vi "Cycle_History_Parse.vi"(10 "Data":string, 11 "Cycle diag in":T1) -> (3 "Cycle diag Out":T1)   [LabVIEW 2014]
uses:
  type defs/Cycle_Diag.ctl
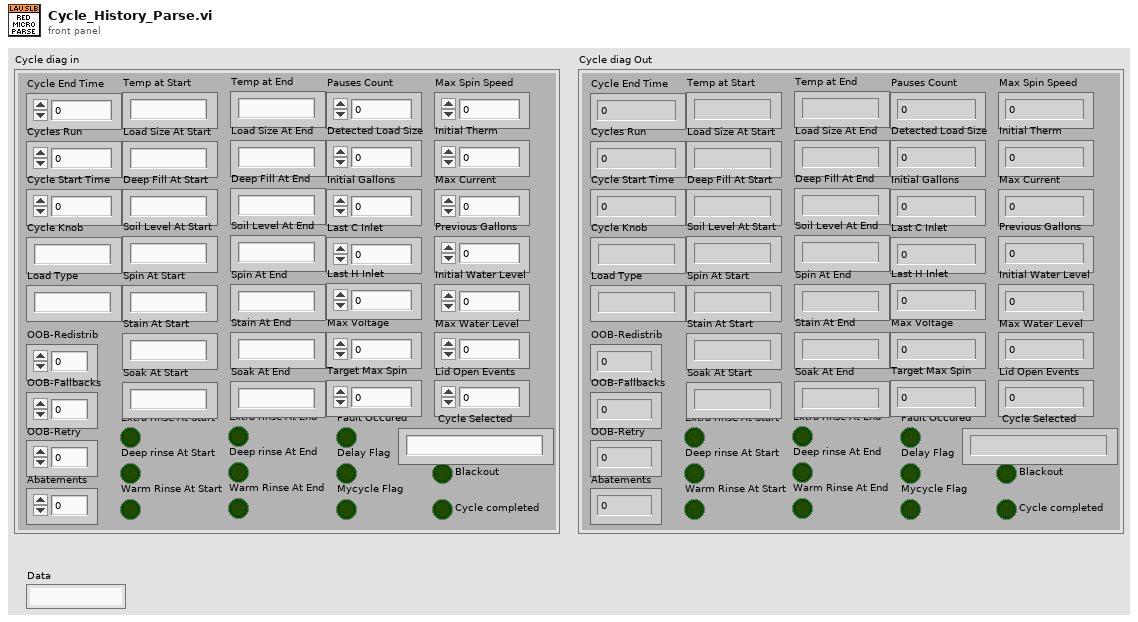
[diagram p1: front panel]
types:
  T1 = typedef "Cycle_Diag.ctl" = cluster{"Cycle End Time":u32, "Cycles Run":u32, "Cycle Start Time":u32, "Cycle Knob":string, "Load Type":string, "OOB-Redistrib":u8, "OOB-Fallbacks":u8, "OOB-Retry":u8, "Temp at Start":string, "Load Size At Start":string, "Deep Fill At Start":string, "Soil Level At Start":string, "Spin At Start":string, "Extra rinse At Start":bool, "Deep rinse At Start":bool, "Stain At Start":string, "Soak At Start":string, "Warm Rinse At Start":bool, "Temp at End":string, "Load Size At End":string, "Deep Fill At End":string, "Soil Level At End":string, "Spin At End":string, "Extra rinse At End":bool, "Deep rinse At End":bool, "Stain At End":string, "Soak At End":string, "Warm Rinse At End":bool, "Pauses Count":u8, "Fault Occured":bool, "Delay Flag":bool, "Mycycle Flag":bool, "Blackout":bool, "Cycle completed":bool, "Detected Load Size":dbl, "Initial Gallons":dbl, "Last C Inlet ":dbl, "Max Voltage":dbl, "Target Max Spin":u16, "Max Spin Speed":u16, "Initial Therm":dbl, "Max Current":dbl, "Previous Gallons":dbl, "Initial Water Level":dbl, "Max Water Level":dbl, "Abatements ":u8, "Lid Open Events":u8, "Cycle Selected":string, "Last H Inlet ":dbl}
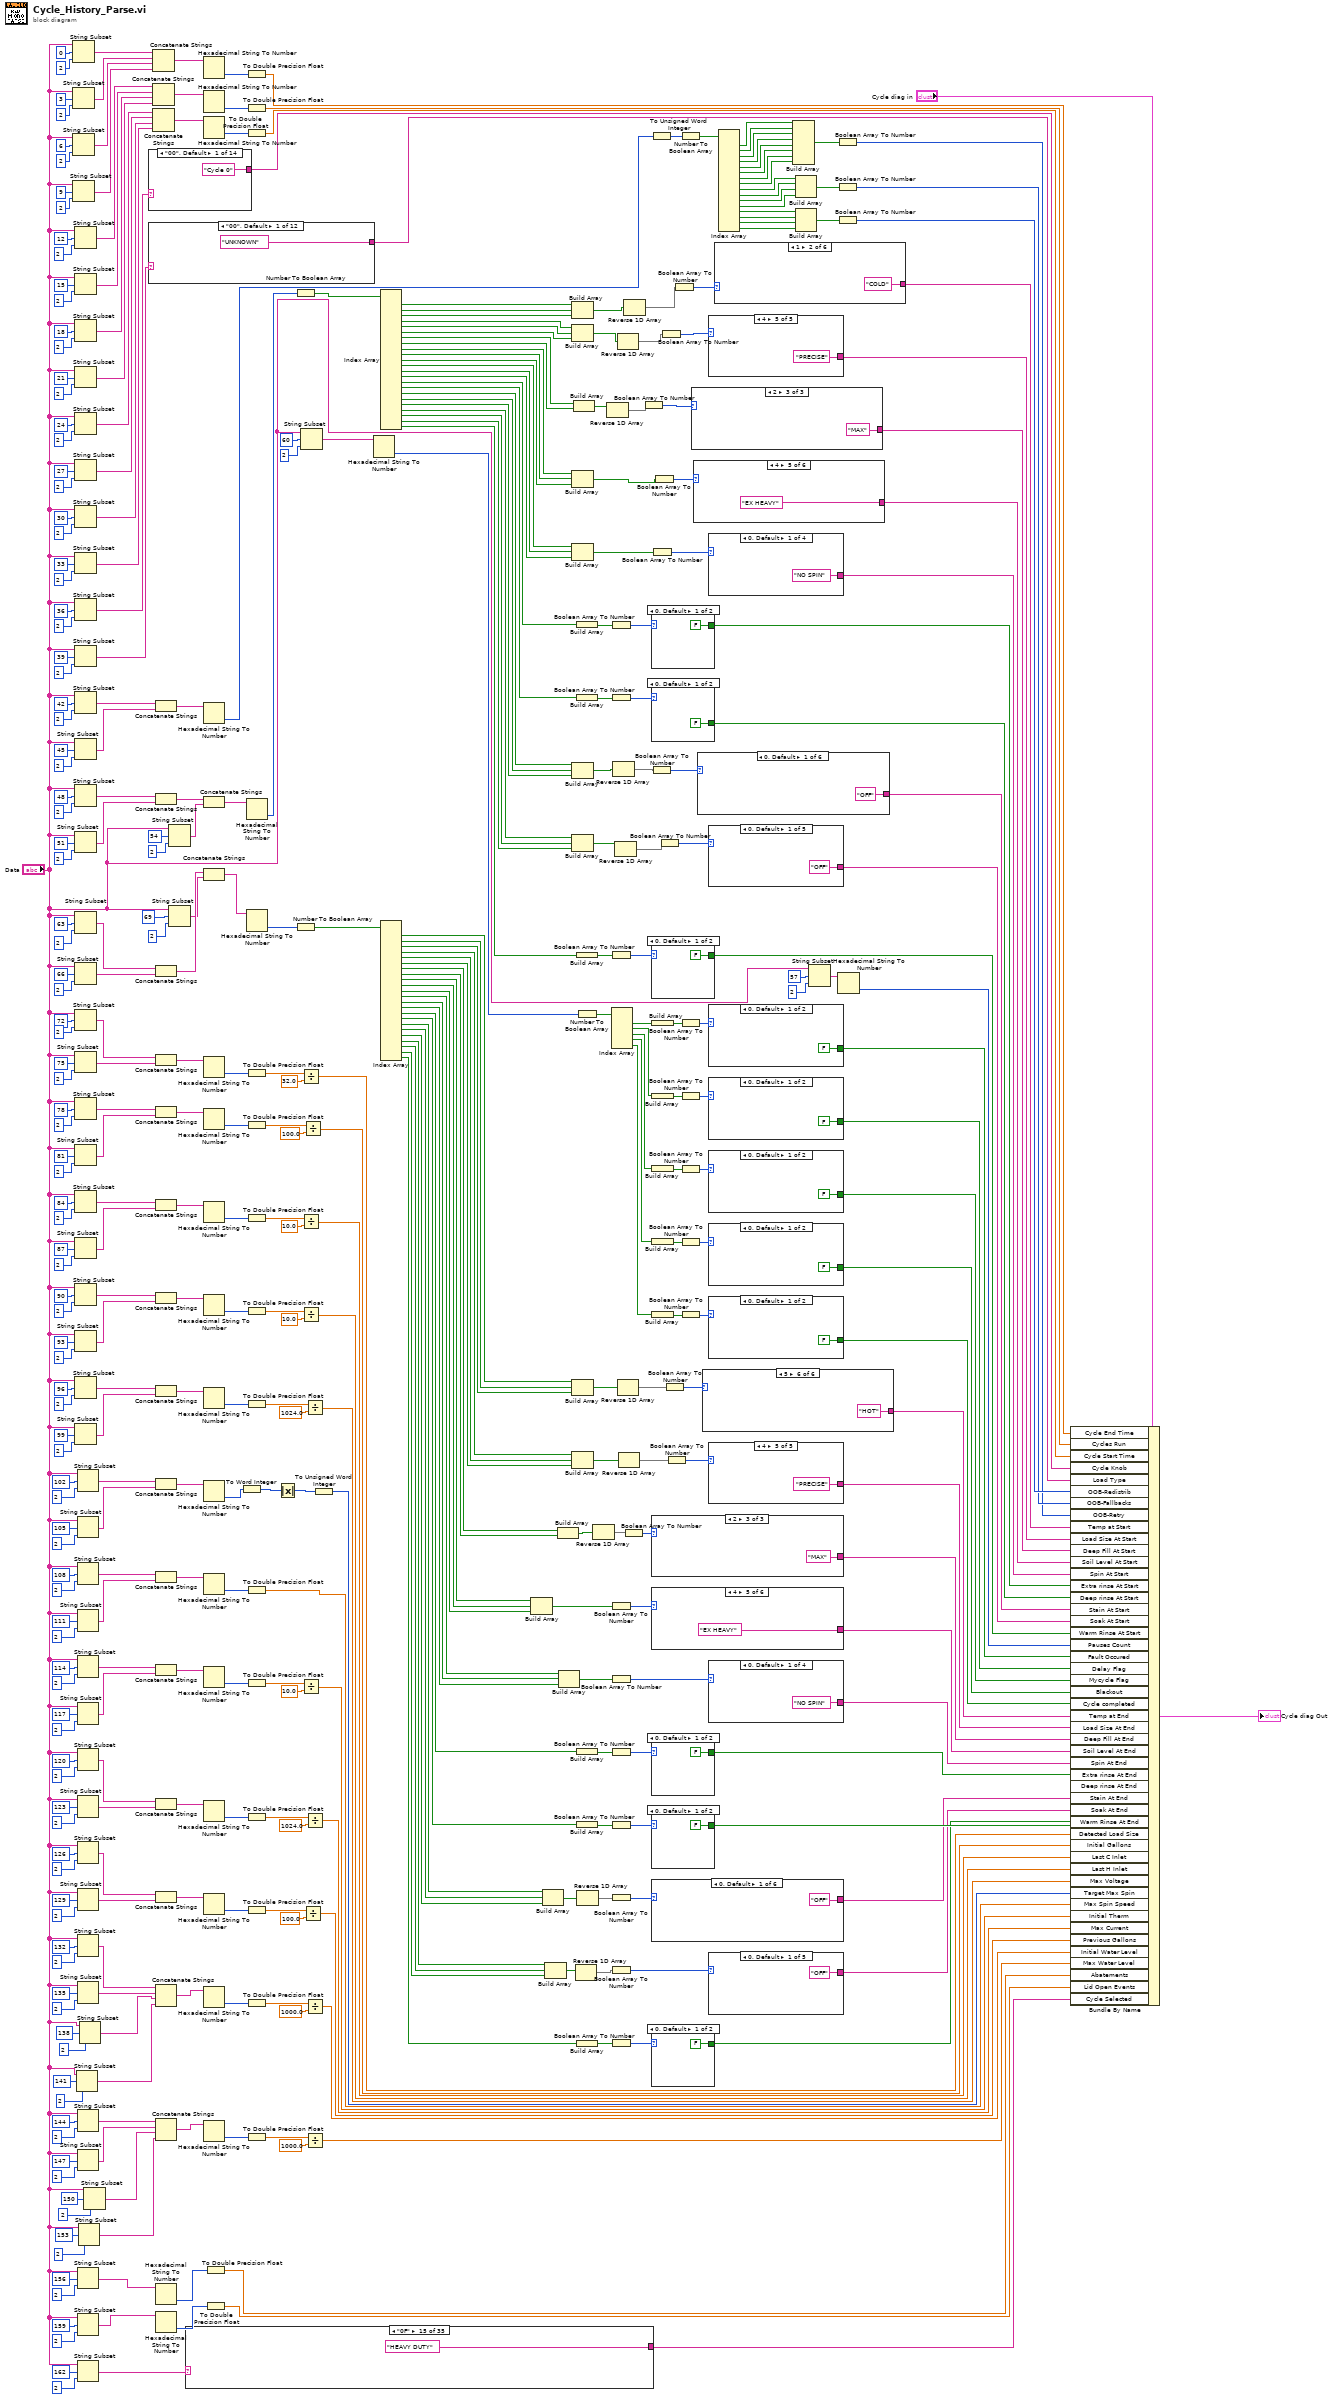
[diagram p0: block diagram]
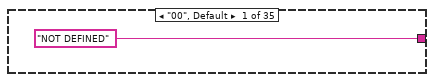
[diagram p2: hidden frame]
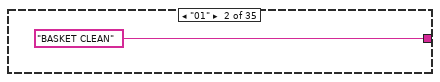
[diagram p3: hidden frame]
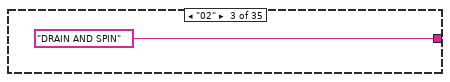
[diagram p4: hidden frame]
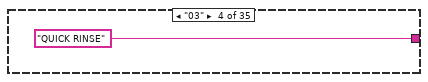
[diagram p5: hidden frame]
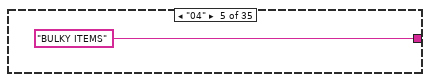
[diagram p6: hidden frame]
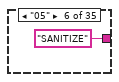
[diagram p7: hidden frame]
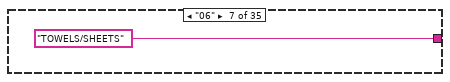
[diagram p8: hidden frame]
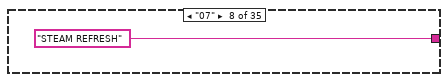
[diagram p9: hidden frame]
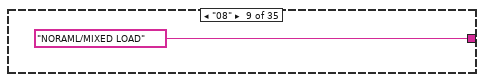
[diagram p10: hidden frame]
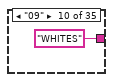
[diagram p11: hidden frame]
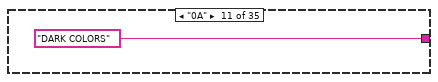
[diagram p12: hidden frame]
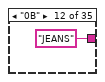
[diagram p13: hidden frame]
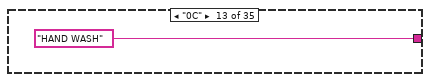
[diagram p14: hidden frame]
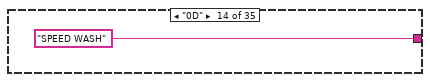
[diagram p15: hidden frame]
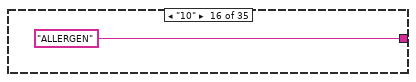
[diagram p16: hidden frame]
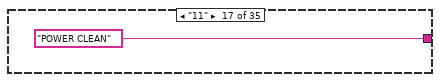
[diagram p17: hidden frame]
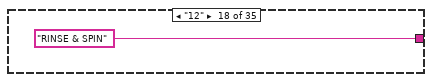
[diagram p18: hidden frame]
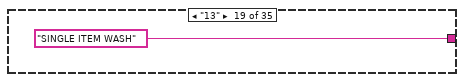
[diagram p19: hidden frame]
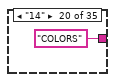
[diagram p20: hidden frame]
diagram:
  n1 = String Subset(string="Data", offset (0)=0, length (rest)=2 ("length (rest)")) -> (substring=w383:string)
  n2 = String Subset(string="Data", offset (0)=3, length (rest)=2 ("length (rest)")) -> (substring=w382:string)
  n3 = String Subset(string="Data", offset (0)=6, length (rest)=2 ("length (rest)")) -> (substring=w381:string)
  n4 = String Subset(string="Data", offset (0)=9, length (rest)=2 ("length (rest)")) -> (substring=w380:string)
  n5 = String Subset(string="Data", offset (0)=12, length (rest)=2 ("length (rest)")) -> (substring=w376:string)
  n6 = String Subset(string="Data", offset (0)=15, length (rest)=2 ("length (rest)")) -> (substring=w375:string)
  n7 = String Subset(string="Data", offset (0)=18, length (rest)=2 ("length (rest)")) -> (substring=w374:string)
  n8 = String Subset(string="Data", offset (0)=21, length (rest)=2 ("length (rest)")) -> (substring=w373:string)
  n9 = String Subset(string="Data", offset (0)=24, length (rest)=2 ("length (rest)")) -> (substring=w369:string)
  n10 = String Subset(string="Data", offset (0)=27, length (rest)=2 ("length (rest)")) -> (substring=w368:string)
  n11 = String Subset(string="Data", offset (0)=30, length (rest)=2 ("length (rest)")) -> (substring=w367:string)
  n12 = String Subset(string="Data", offset (0)=33, length (rest)=2 ("length (rest)")) -> (substring=w366:string)
  n13 = String Subset(string="Data", offset (0)=36, length (rest)=2 ("length (rest)")) -> (substring=w362:string)
  n14 = String Subset(string="Data", offset (0)=39, length (rest)=2 ("length (rest)")) -> (substring=w360:string)
  n15 = String Subset(string="Data", offset (0)=42, length (rest)=2 ("length (rest)")) -> (substring=w358:string)
  n16 = String Subset(string="Data", offset (0)=45, length (rest)=2 ("length (rest)")) -> (substring=w357:string)
  n17 = String Subset(string="Data", offset (0)=48, length (rest)=2 ("length (rest)")) -> (substring=w322:string)
  n18 = String Subset(string="Data", offset (0)=51, length (rest)=2 ("length (rest)")) -> (substring=w321:string)
  n19 = String Subset(string="Data", offset (0)=63, length (rest)=2 ("length (rest)")) -> (substring=w264:string)
  n20 = String Subset(string="Data", offset (0)=66, length (rest)=2 ("length (rest)")) -> (substring=w263:string)
  n21 = String Subset(string="Data", offset (0)=72, length (rest)=2 ("length (rest)")) -> (substring=w175:string)
  n22 = String Subset(string="Data", offset (0)=75 ("offset"), length (rest)=u32 2 ("default (0 U32)")) -> (substring=w172:string)
  n23 = String Subset(string="Data", offset (0)=78, length (rest)=2 ("length (rest)")) -> (substring=w167:string)
  n24 = String Subset(string="Data", offset (0)=81, length (rest)=2 ("length (rest)")) -> (substring=w166:string)
  n25 = String Subset(string="Data", offset (0)=84, length (rest)=2 ("length (rest)")) -> (substring=w155:string)
  n26 = String Subset(string="Data", offset (0)=87, length (rest)=2 ("length (rest)")) -> (substring=w154:string)
  n27 = String Subset(string="Data", offset (0)=90, length (rest)=2 ("length (rest)")) -> (substring=w148:string)
  n28 = String Subset(string="Data", offset (0)=93, length (rest)=2 ("length (rest)")) -> (substring=w147:string)
  n29 = String Subset(string="Data", offset (0)=96, length (rest)=2 ("length (rest)")) -> (substring=w137:string)
  n30 = String Subset(string="Data", offset (0)=99, length (rest)=2 ("length (rest)")) -> (substring=w136:string)
  n31 = String Subset(string="Data", offset (0)=141, length (rest)=2 ("length (rest)")) -> (substring=w41:string)
  n32 = String Subset(string="Data", offset (0)=102, length (rest)=2 ("length (rest)")) -> (substring=w126:string)
  n33 = String Subset(string="Data", offset (0)=105, length (rest)=2 ("length (rest)")) -> (substring=w125:string)
  n34 = String Subset(string="Data", offset (0)=108, length (rest)=2 ("length (rest)")) -> (substring=w123:string)
  n35 = String Subset(string="Data", offset (0)=111, length (rest)=2 ("length (rest)")) -> (substring=w122:string)
  n36 = String Subset(string="Data", offset (0)=114, length (rest)=2 ("length (rest)")) -> (substring=w111:string)
  n37 = String Subset(string="Data", offset (0)=117, length (rest)=2 ("length (rest)")) -> (substring=w110:string)
  n38 = String Subset(string="Data", offset (0)=120, length (rest)=2 ("length (rest)")) -> (substring=w100:string)
  n39 = String Subset(string="Data", offset (0)=123, length (rest)=2 ("length (rest)")) -> (substring=w99:string)
  n40 = String Subset(string="Data", offset (0)=126, length (rest)=2 ("length (rest)")) -> (substring=w89:string)
  n41 = String Subset(string="Data", offset (0)=129, length (rest)=2 ("length (rest)")) -> (substring=w88:string)
  n42 = String Subset(string="Data", offset (0)=132, length (rest)=2 ("length (rest)")) -> (substring=w78:string)
  n43 = String Subset(string="Data", offset (0)=135, length (rest)=2 ("length (rest)")) -> (substring=w77:string)
  n44 = String Subset(string="Data", offset (0)=144, length (rest)=2 ("length (rest)")) -> (substring=w72:string)
  n45 = String Subset(string="Data", offset (0)=147, length (rest)=2 ("length (rest)")) -> (substring=w71:string)
  n46 = String Subset(string="Data", offset (0)=156, length (rest)=2 ("length (rest)")) -> (substring=w50:string)
  n47 = String Subset(string="Data", offset (0)=159, length (rest)=2 ("length (rest)")) -> (substring=w49:string)
  n48 = String Subset(string="Data", offset (0)=162, length (rest)=2 ("length (rest)")) -> (substring=w44:string)
  n49 = String Subset(string="Data", offset (0)=153, length (rest)=2 ("length (rest)")) -> (substring=w35:string)
  n50 = String Subset(string="Data", offset (0)=138, length (rest)=2 ("length (rest)")) -> (substring=w42:string)
  n51 = String Subset(string="Data", offset (0)=150, length (rest)=2 ("length (rest)")) -> (substring=w36:string)
  n52 = case shown="\"00\", Default" w362 {
    tunnel: ["Cycle 0" "Cycle 1" "Cycle 2" "Cycle 3" "Cycle 4" "Cycle 5" "Cycle 6" "Cycle 7" "Cycle 8" "Cycle 9" "Cycle 10" "Cycle 11" "Cycle 12" "Cycle 13"] -> w361
    frame "00", Default {
    }
    frame "01" {
    }
    frame "02" {
    }
    frame "03" {
    }
    frame "04" {
    }
    frame "05" {
    }
    frame "06" {
    }
    frame "07" {
    }
    frame "08" {
    }
    frame "09" {
    }
    frame "0A" {
    }
    frame "0B" {
    }
    frame "0C" {
    }
    frame "0D" {
    }
  }
  n53 = case shown="\"00\", Default" w360 {
    tunnel: ["UNKNOWN" "COTTON" "SYNTHETIC" "MIXED" "WET" "LOW FLOW" "SMALL" "MEDIUM" "LARGE" "SUPER" "SUPER PLUS" "MAX"] -> w359
    frame "00", Default {
    }
    frame "01" {
    }
    frame "02" {
    }
    frame "03" {
    }
    frame "04" {
    }
    frame "05" {
    }
    frame "06" {
    }
    frame "07" {
    }
    frame "08" {
    }
    frame "09" {
    }
    frame "0A" {
    }
    frame "0B" {
    }
  }
  n54 = Concatenate Strings(w383, w382, w381, w380) -> (w379:string)
  n55 = Concatenate Strings(w376, w375, w374, w373) -> (w372:string)
  n56 = Concatenate Strings(w369, w368, w367, w366) -> (w365:string)
  n57 = Concatenate Strings(w358, w357) -> (w356:string)
  n58 = Concatenate Strings(w322, w321) -> (w320:string)
  n59 = Concatenate Strings(w264, w263) -> (w262:string)
  n60 = Concatenate Strings(w175, w172) -> (w171:string)
  n61 = Concatenate Strings(w167, w166) -> (w165:string)
  n62 = Concatenate Strings(w155, w154) -> (w153:string)
  n63 = Concatenate Strings(w148, w147) -> (w146:string)
  n64 = Concatenate Strings(w137, w136) -> (w135:string)
  n65 = Concatenate Strings(w126, w125) -> (w124:string)
  n66 = Concatenate Strings(w123, w122) -> (w121:string)
  n67 = Concatenate Strings(w111, w110) -> (w109:string)
  n68 = Concatenate Strings(w100, w99) -> (w98:string)
  n69 = Concatenate Strings(w89, w88) -> (w87:string)
  n70 = Concatenate Strings(w78, w77, w42, w41) -> (w76:string)
  n71 = Concatenate Strings(w72, w71, w36, w35) -> (w70:string)
  n72 = Hexadecimal String To Number(string=w50) -> (number=w48:u32)  [unwired: 2 in, 1 out]
  n73 = Hexadecimal String To Number(string=w49) -> (number=w47:u32)  [unwired: 2 in, 1 out]
  n74 = String Subset(string="Data", offset (0)=54, length (rest)=2 ("length (rest)")) -> (substring=w319:string)
  n75 = String Subset(string="Data", offset (0)=69, length (rest)=2 ("length (rest)")) -> (substring=w261:string)
  n76 = case shown="\"0F\"" w44 {
    tunnel: ["NOT DEFINED" "BASKET CLEAN" "DRAIN AND SPIN" "QUICK RINSE" "BULKY ITEMS" "SANITIZE" "TOWELS/SHEETS" "STEAM REFRESH" "NORAML/MIXED LOAD" "WHITES" "DARK COLORS" "JEANS" "HAND WASH" "SPEED WASH" "HEAVY DUTY" "ALLERGEN" "POWER CLEAN" "RINSE & SPIN" "SINGLE ITEM WASH" "COLORS" "COLD WASH" "COTTONS" "EASY CARE" "ACTIVE WEAR" "TIMED DRY" "DEWRINKLE" "QUICK/AIR FLUFF" "STEAM REFRESH" "STEAM DEWRINKLE" "SPEED DRY" "MIXED" "QUICK DRY" "CASUALS" "WARM UP" "ENERGY SAVER"] -> w43
    frame "00", Default {
    }
    frame "01" {
    }
    frame "02" {
    }
    frame "03" {
    }
    frame "04" {
    }
    frame "05" {
    }
    frame "06" {
    }
    frame "07" {
    }
    frame "08" {
    }
    frame "09" {
    }
    frame "0A" {
    }
    frame "0B" {
    }
    frame "0C" {
    }
    frame "0D" {
    }
    frame "0F" {
    }
    frame "10" {
    }
    frame "11" {
    }
    frame "12" {
    }
    frame "13" {
    }
    frame "14" {
    }
    frame "15" {
    }
    frame "80" {
    }
    frame "81" {
    }
    frame "82" {
    }
    frame "83" {
    }
    frame "84" {
    }
    frame "85" {
    }
    frame "86" {
    }
    frame "87" {
    }
    frame "88" {
    }
    frame "89" {
    }
    frame "8A" {
    }
    frame "8B" {
    }
    frame "8C" {
    }
    frame "8D" {
    }
  }
  n77 = Hexadecimal String To Number(string=w379) -> (number=w378:u32)  [unwired: 2 in, 1 out]
  n78 = Hexadecimal String To Number(string=w372) -> (number=w371:u32)  [unwired: 2 in, 1 out]
  n79 = Hexadecimal String To Number(string=w365) -> (number=w364:u32)  [unwired: 2 in, 1 out]
  n80 = Hexadecimal String To Number(string=w356) -> (number=w353:u32)  [unwired: 2 in, 1 out]
  n81 = Concatenate Strings(w320, w319) -> (w318:string)
  n82 = Concatenate Strings(w262, w261) -> (w260:string)
  n83 = Hexadecimal String To Number(string=w171) -> (number=w179:u32)  [unwired: 2 in, 1 out]
  n84 = Hexadecimal String To Number(string=w165) -> (number=w164:u32)  [unwired: 2 in, 1 out]
  n85 = Hexadecimal String To Number(string=w153) -> (number=w152:u32)  [unwired: 2 in, 1 out]
  n86 = Hexadecimal String To Number(string=w146) -> (number=w145:u32)  [unwired: 2 in, 1 out]
  n87 = Hexadecimal String To Number(string=w135) -> (number=w134:u32)  [unwired: 2 in, 1 out]
  n88 = Hexadecimal String To Number(string=w124) -> (number=w26:u32)  [unwired: 2 in, 1 out]
  n89 = Hexadecimal String To Number(string=w121) -> (number=w120:u32)  [unwired: 2 in, 1 out]
  n90 = Hexadecimal String To Number(string=w109) -> (number=w108:u32)  [unwired: 2 in, 1 out]
  n91 = Hexadecimal String To Number(string=w98) -> (number=w97:u32)  [unwired: 2 in, 1 out]
  n92 = Hexadecimal String To Number(string=w87) -> (number=w86:u32)  [unwired: 2 in, 1 out]
  n93 = Hexadecimal String To Number(string=w76) -> (number=w75:u32)  [unwired: 2 in, 1 out]
  n94 = Hexadecimal String To Number(string=w70) -> (number=w69:u32)  [unwired: 2 in, 1 out]
  n95 = To Double Precision Float(number=w48) -> (double precision float=w46:dbl)
  n96 = To Double Precision Float(number=w47) -> (double precision float=w45:dbl)
  n97 = To Word Integer(number=w26) -> (16bit integer=w28:i16)
  n98 = To Double Precision Float(number=w378) -> (double precision float=w377:dbl)
  n99 = To Double Precision Float(number=w371) -> (double precision float=w370:dbl)
  n100 = To Double Precision Float(number=w364) -> (double precision float=w363:dbl)
  n101 = Hexadecimal String To Number(string=w318) -> (number=w317:u32)  [unwired: 2 in, 1 out]
  n102 = Hexadecimal String To Number(string=w260) -> (number=w259:u32)  [unwired: 2 in, 1 out]
  n103 = To Double Precision Float(number=w179) -> (double precision float=w178:dbl)
  n104 = To Double Precision Float(number=w164) -> (double precision float=w163:dbl)
  n105 = To Double Precision Float(number=w152) -> (double precision float=w151:dbl)
  n106 = To Double Precision Float(number=w145) -> (double precision float=w144:dbl)
  n107 = To Double Precision Float(number=w134) -> (double precision float=w133:dbl)
  n108 = To Double Precision Float(number=w120) -> (double precision float=w29:dbl)
  n109 = To Double Precision Float(number=w108) -> (double precision float=w107:dbl)
  n110 = To Double Precision Float(number=w97) -> (double precision float=w96:dbl)
  n111 = To Double Precision Float(number=w86) -> (double precision float=w85:dbl)
  n112 = To Double Precision Float(number=w75) -> (double precision float=w74:dbl)
  n113 = To Double Precision Float(number=w69) -> (double precision float=w68:dbl)
  n114 = Absolute Value(x=w28) -> (abs(x)=w27:i16)
  n115 = Number To Boolean Array(number=w317) -> (Boolean array=w316:bool[])
  n116 = Number To Boolean Array(number=w259) -> (Boolean array=w225:bool[])
  n117 = String Subset(string="Data", offset (0)=60, length (rest)=2 ("length (rest)")) -> (substring=w204:string)
  n118 = Divide(x=w178, y=32.0) -> (x/y=w176:dbl)
  n119 = Divide(x=w151, y=10.0) -> (x/y=w149:dbl)
  n120 = Divide(x=w144, y=10.0) -> (x/y=w138:dbl)
  n121 = Divide(x=w107, y=10.0) -> (x/y=w101:dbl)
  n122 = Divide(x=w163, y=100.0) -> (x/y=w161:dbl)
  n123 = Divide(x=w85, y=100.0) -> (x/y=w79:dbl)
  n124 = Divide(x=w133, y=1024.0) -> (x/y=w127:dbl)
  n125 = Divide(x=w96, y=1024.0) -> (x/y=w90:dbl)
  n126 = Divide(x=w74, y=1000.0) -> (x/y=w58:dbl)
  n127 = Divide(x=w68, y=1000.0) -> (x/y=w57:dbl)
  n128 = To Unsigned Word Integer(number=w27) -> (unsigned 16bit integer=w25:u16)
  n129 = Hexadecimal String To Number(string=w204) -> (number=w203:u32)  [unwired: 2 in, 1 out]
  n130 = Index Array(array=w316) -> (element #1=w315:bool, element #2=w314:bool, element #3=w313:bool, element #4=w312:bool, element #5=w311:bool, element #6=w310:bool, element #7=w309:bool, element #8=w308:bool, element #9=w307:bool, element #10=w306:bool, element #11=w305:bool, element #12=w304:bool, element #13=w303:bool, element #14=w302:bool, element #15=w301:bool, element #16=w300:bool, element #17=w299:bool, element #18=w298:bool, element #19=w297:bool, element #20=w296:bool, element #21=w295:bool, element #22=w294:bool, element #23=w293:bool)  [unwired: 23 in]
  n131 = Index Array(array=w225) -> (element #1=w258:bool, element #2=w257:bool, element #3=w256:bool, element #4=w255:bool, element #5=w254:bool, element #6=w253:bool, element #7=w252:bool, element #8=w251:bool, element #9=w250:bool, element #10=w249:bool, element #11=w248:bool, element #12=w247:bool, element #13=w246:bool, element #14=w245:bool, element #15=w244:bool, element #16=w243:bool, element #17=w242:bool, element #18=w241:bool, element #19=w240:bool, element #20=w239:bool, element #21=w238:bool, element #22=w237:bool, element #23=w236:bool)  [unwired: 23 in]
  n132 = Build Array(w250, w249, w248) -> (w7:bool[])
  n133 = Build Array(w242, w241, w240) -> (w4:bool[])
  n134 = Build Array(w239, w238, w237) -> (w2:bool[])
  n135 = Build Array(w252, w251) -> (w8:bool[])
  n136 = Build Array(w247, w246, w245) -> (w224:bool[])
  n137 = Build Array(w315, w314, w313) -> (w24:bool[])
  n138 = Build Array(w312, w311, w310) -> (w21:bool[])
  n139 = Build Array(w307, w306, w305) -> (w5:bool[])
  n140 = Build Array(w304, w303, w302) -> (w6:bool[])
  n141 = Build Array(w299, w298, w297) -> (w17:bool[])
  n142 = Build Array(w296, w295, w294) -> (w15:bool[])
  n143 = Build Array(w258, w257, w256) -> (w12:bool[])
  n144 = Build Array(w255, w254, w253) -> (w11:bool[])
  n145 = Build Array(w309, w308) -> (w19:bool[])
  n146 = Reverse 1D Array(array=w2) -> (reversed array=w1:bool[])
  n147 = Build Array(w301) -> (w283:bool[])
  n148 = Build Array(w300) -> (w282:bool[])
  n149 = Build Array(w293) -> (w273:bool[])
  n150 = Build Array(w244) -> (w223:bool[])
  n151 = Build Array(w243) -> (w222:bool[])
  n152 = Build Array(w236) -> (w221:bool[])
  n153 = Number To Boolean Array(number=w203) -> (Boolean array=w202:bool[])
  n154 = Reverse 1D Array(array=w4) -> (reversed array=w3:bool[])
  n155 = Reverse 1D Array(array=w8) -> (reversed array=w9:bool[])
  n156 = Reverse 1D Array(array=w19) -> (reversed array=w18:bool[])
  n157 = Boolean Array To Number(Boolean array=w283) -> (number=w281:u32)
  n158 = Boolean Array To Number(Boolean array=w282) -> (number=w280:u32)
  n159 = Boolean Array To Number(Boolean array=w273) -> (number=w272:u32)
  n160 = Boolean Array To Number(Boolean array=w7) -> (number=w232:u32)
  n161 = Boolean Array To Number(Boolean array=w224) -> (number=w231:u32)
  n162 = Boolean Array To Number(Boolean array=w223) -> (number=w230:u32)
  n163 = Boolean Array To Number(Boolean array=w222) -> (number=w229:u32)
  n164 = Boolean Array To Number(Boolean array=w3) -> (number=w228:u32)
  n165 = Boolean Array To Number(Boolean array=w1) -> (number=w227:u32)
  n166 = Boolean Array To Number(Boolean array=w221) -> (number=w226:u32)
  n167 = Index Array(array=w202) -> (element #1=w201:bool, element #2=w200:bool, element #3=w199:bool, element #4=w198:bool, element #5=w197:bool)  [unwired: 5 in]
  n168 = Reverse 1D Array(array=w17) -> (reversed array=w16:bool[])
  n169 = Reverse 1D Array(array=w15) -> (reversed array=w14:bool[])
  n170 = Reverse 1D Array(array=w21) -> (reversed array=w20:bool[])
  n171 = Reverse 1D Array(array=w12) -> (reversed array=w13:bool[])
  n172 = Reverse 1D Array(array=w11) -> (reversed array=w10:bool[])
  n173 = Boolean Array To Number(Boolean array=w9) -> (number=w233:u32)
  n174 = Reverse 1D Array(array=w24) -> (reversed array=w23:bool[])
  n175 = Boolean Array To Number(Boolean array=w18) -> (number=w289:u32)
  n176 = To Unsigned Word Integer(number=w353) -> (unsigned 16bit integer=w352:u16)
  n177 = Boolean Array To Number(Boolean array=w16) -> (number=w277:u32)
  n178 = Boolean Array To Number(Boolean array=w6) -> (number=w285:u32)
  n179 = case shown="0, Default" w281 {
    tunnel: [FALSE TRUE] -> w279
    frame 0, Default {
    }
    frame 1 {
    }
  }
  n180 = case shown="0, Default" w280 {
    tunnel: [FALSE TRUE] -> w278
    frame 0, Default {
    }
    frame 1 {
    }
  }
  n181 = case shown="0, Default" w272 {
    tunnel: [FALSE TRUE] -> w271
    frame 0, Default {
    }
    frame 1 {
    }
  }
  n182 = Build Array(w201) -> (w192:bool[])
  n183 = Build Array(w200) -> (w193:bool[])
  n184 = Build Array(w199) -> (w194:bool[])
  n185 = Build Array(w198) -> (w195:bool[])
  n186 = Build Array(w197) -> (w196:bool[])
  n187 = case shown="2" w233 {
    tunnel: ["OFF" "INCREMENTAL" "MAX"] -> w218
    frame 0, Default {
    }
    frame 1 {
    }
    frame 2 {
    }
  }
  n188 = case shown="4" w232 {
    tunnel: ["EXTRA LIGHT" "LIGHT" "NORMAL" "HEAVY" "EX HEAVY" "DISABLED"] -> w217
    frame 0, Default {
    }
    frame 1 {
    }
    frame 2 {
    }
    frame 3 {
    }
    frame 4 {
    }
    frame 5 {
    }
  }
  n189 = case shown="0, Default" w230 {
    tunnel: [FALSE TRUE] -> w215
    frame 0, Default {
    }
    frame 1 {
    }
  }
  n190 = case shown="0, Default" w229 {
    tunnel: [FALSE TRUE] -> w214
    frame 0, Default {
    }
    frame 1 {
    }
  }
  n191 = case shown="0, Default" w228 {
    tunnel: ["OFF" "TOMATO" "WINE" "BLOOD" "GRASS" "DIRT"] -> w213
    frame 0, Default {
    }
    frame 1 {
    }
    frame 2 {
    }
    frame 3 {
    }
    frame 4 {
    }
    frame 5 {
    }
  }
  n192 = case shown="0, Default" w226 {
    tunnel: [FALSE TRUE] -> w211
    frame 0, Default {
    }
    frame 1 {
    }
  }
  n193 = Boolean Array To Number(Boolean array=w5) -> (number=w287:u32)
  n194 = Boolean Array To Number(Boolean array=w14) -> (number=w275:u32)
  n195 = Boolean Array To Number(Boolean array=w20) -> (number=w291:u32)
  n196 = Boolean Array To Number(Boolean array=w13) -> (number=w235:u32)
  n197 = Boolean Array To Number(Boolean array=w10) -> (number=w234:u32)
  n198 = Boolean Array To Number(Boolean array=w23) -> (number=w22:u32)
  n199 = Number To Boolean Array(number=w352) -> (Boolean array=w345:bool[])
  n200 = Boolean Array To Number(Boolean array=w192) -> (number=w191:u32)
  n201 = Boolean Array To Number(Boolean array=w193) -> (number=w190:u32)
  n202 = Boolean Array To Number(Boolean array=w194) -> (number=w189:u32)
  n203 = Boolean Array To Number(Boolean array=w195) -> (number=w188:u32)
  n204 = Boolean Array To Number(Boolean array=w196) -> (number=w187:u32)
  n205 = case shown="2" w289 {
    tunnel: ["OFF" "INCREMENTAL" "MAX"] -> w288
    frame 0, Default {
    }
    frame 1 {
    }
    frame 2 {
    }
  }
  n206 = case shown="4" w287 {
    tunnel: ["EXTRA LIGHT" "LIGHT" "NORMAL" "HEAVY" "EX HEAVY" "DISABLED"] -> w286
    frame 0, Default {
    }
    frame 1 {
    }
    frame 2 {
    }
    frame 3 {
    }
    frame 4 {
    }
    frame 5 {
    }
  }
  n207 = case shown="0, Default" w277 {
    tunnel: ["OFF" "TOMATO" "WINE" "BLOOD" "GRASS" "DIRT"] -> w276
    frame 0, Default {
    }
    frame 1 {
    }
    frame 2 {
    }
    frame 3 {
    }
    frame 4 {
    }
    frame 5 {
    }
  }
  n208 = case shown="5" w235 {
    tunnel: ["TAP COLD" "COLD" "COOL" "COLORS" "WARM" "HOT"] -> w220
    frame 0, Default {
    }
    frame 1 {
    }
    frame 2 {
    }
    frame 3 {
    }
    frame 4 {
    }
    frame 5 {
    }
  }
  n209 = case shown="4" w291 {
    tunnel: ["SMALL" "MEDIUM" "LARGE" "SUPER" "PRECISE"] -> w290
    frame 0, Default {
    }
    frame 1 {
    }
    frame 2 {
    }
    frame 3 {
    }
    frame 4 {
    }
  }
  n210 = case shown="0, Default" w285 {
    tunnel: ["NO SPIN" "NORMAL" "MORE" "MAX"] -> w284
    frame 0, Default {
    }
    frame 1 {
    }
    frame 2 {
    }
    frame 3 {
    }
  }
  n211 = case shown="0, Default" w275 {
    tunnel: ["OFF" "15 MIN" "30 MIN" "60 MIN" "2 HOURS"] -> w274
    frame 0, Default {
    }
    frame 1 {
    }
    frame 2 {
    }
    frame 3 {
    }
    frame 4 {
    }
  }
  n212 = case shown="0, Default" w191 {
    tunnel: [FALSE TRUE] -> w186
    frame 0, Default {
    }
    frame 1 {
    }
  }
  n213 = case shown="0, Default" w190 {
    tunnel: [FALSE TRUE] -> w185
    frame 0, Default {
    }
    frame 1 {
    }
  }
  n214 = case shown="0, Default" w189 {
    tunnel: [FALSE TRUE] -> w184
    frame 0, Default {
    }
    frame 1 {
    }
  }
  n215 = case shown="0, Default" w188 {
    tunnel: [FALSE TRUE] -> w183
    frame 0, Default {
    }
    frame 1 {
    }
  }
  n216 = case shown="0, Default" w187 {
    tunnel: [FALSE TRUE] -> w182
    frame 0, Default {
    }
    frame 1 {
    }
  }
  n217 = case shown="4" w234 {
    tunnel: ["SMALL" "MEDIUM" "LARGE" "SUPER" "PRECISE"] -> w219
    frame 0, Default {
    }
    frame 1 {
    }
    frame 2 {
    }
    frame 3 {
    }
    frame 4 {
    }
  }
  n218 = case shown="0, Default" w231 {
    tunnel: ["NO SPIN" "NORMAL" "MORE" "MAX"] -> w216
    frame 0, Default {
    }
    frame 1 {
    }
    frame 2 {
    }
    frame 3 {
    }
  }
  n219 = case shown="0, Default" w227 {
    tunnel: ["OFF" "15 MIN" "30 MIN" "60 MIN" "2 HOURS"] -> w212
    frame 0, Default {
    }
    frame 1 {
    }
    frame 2 {
    }
    frame 3 {
    }
    frame 4 {
    }
  }
  n220 = case shown="1" w22 {
    tunnel: ["TAP COLD" "COLD" "COOL" "COLORS" "WARM" "HOT"] -> w292
    frame 0, Default {
    }
    frame 1 {
    }
    frame 2 {
    }
    frame 3 {
    }
    frame 4 {
    }
    frame 5 {
    }
  }
  n221 = Index Array(array=w345) -> (element #1=w344:bool, element #2=w343:bool, element #3=w342:bool, element #4=w341:bool, element #5=w340:bool, element #6=w339:bool, element #7=w338:bool, element #8=w337:bool, element #9=w336:bool, element #10=w335:bool, element #11=w334:bool, element #12=w333:bool, element #13=w332:bool, element #14=w331:bool, element #15=w330:bool, element #16=w329:bool)  [unwired: 16 in]
  n222 = Build Array(w344, w343, w342, w341, w340, w339, w338, w337) -> (w350:bool[])
  n223 = Build Array(w336, w335, w334, w333) -> (w349:bool[])
  n224 = Build Array(w332, w331, w330, w329) -> (w351:bool[])
  n225 = String Subset(string="Data", offset (0)=57, length (rest)=2 ("length (rest)")) -> (substring=w206:string)
  n226 = Boolean Array To Number(Boolean array=w350) -> (number=w346:u32)
  n227 = Boolean Array To Number(Boolean array=w349) -> (number=w347:u32)
  n228 = Boolean Array To Number(Boolean array=w351) -> (number=w348:u32)
  n229 = Hexadecimal String To Number(string=w206) -> (number=w205:u32)  [unwired: 2 in, 1 out]
  n230 = Bundle By Name(cluster="Cycle diag in", "Cycle End Time"=w377, "Cycles Run"=w370, "Cycle Start Time"=w363, "Cycle Knob"=w361, "Load Type"=w359, "OOB-Redistrib"=w348, "OOB-Fallbacks"=w347, "OOB-Retry"=w346, "Temp at Start"=w292, "Load Size At Start"=w290, "Deep Fill At Start"=w288, "Soil Level At Start"=w286, "Spin At Start"=w284, "Extra rinse At Start"=w279, "Deep rinse At Start"=w278, "Stain At Start"=w276, "Soak At Start"=w274, "Warm Rinse At Start"=w271, "Pauses Count"=w205, "Fault Occured"=w186, "Delay Flag"=w185, "Mycycle Flag"=w184, "Blackout"=w183, "Cycle completed"=w182, "Temp at End"=w220, "Load Size At End"=w219, "Deep Fill At End"=w218, "Soil Level At End"=w217, "Spin At End"=w216, "Extra rinse At End"=w215, "Deep rinse At End"=w214, "Stain At End"=w213, "Soak At End"=w212, "Warm Rinse At End"=w211, "Detected Load Size"=w176, "Initial Gallons"=w161, "Last C Inlet"=w149, "Last H Inlet"=w138, "Max Voltage"=w127, "Target Max Spin"=w25, "Max Spin Speed"=w29, "Initial Therm"=w101, "Max Current"=w90, "Previous Gallons"=w79, "Initial Water Level"=w58, "Max Water Level"=w57, "Abatements"=w46, "Lid Open Events"=w45, "Cycle Selected"=w43) -> (→"Cycle diag Out":T1)
